vi "Array to Cluster.vi"() -> ()   [LabVIEW 2018]
doc: "Demonstrates the Array to Cluster function."
panel:
  out "Cluster":T1
  in  "Array of Strings":string[](array[string])=["A", "B", "C", "D", "E", "F"]
  # "Overview: Demonstrates the Array to Cluster function.\nInstructions:\n1. Run the VI to convert a portion of the Array of Strings to a Cluster.\n2. Open the block diagram. Right-click on the Array to Cluster function and select Cluster Size from the menu. Change the cluster size to 6.\n3. The VI is now broken because the Cluster indicator does not have six elements.\n4. Delete the Cluster indicator.\n5. On the block diagram, right-click on the output of the Array to Cluster function and select Create > Indicator from the menu. Remove any broken wires.\n6. Run the VI again."
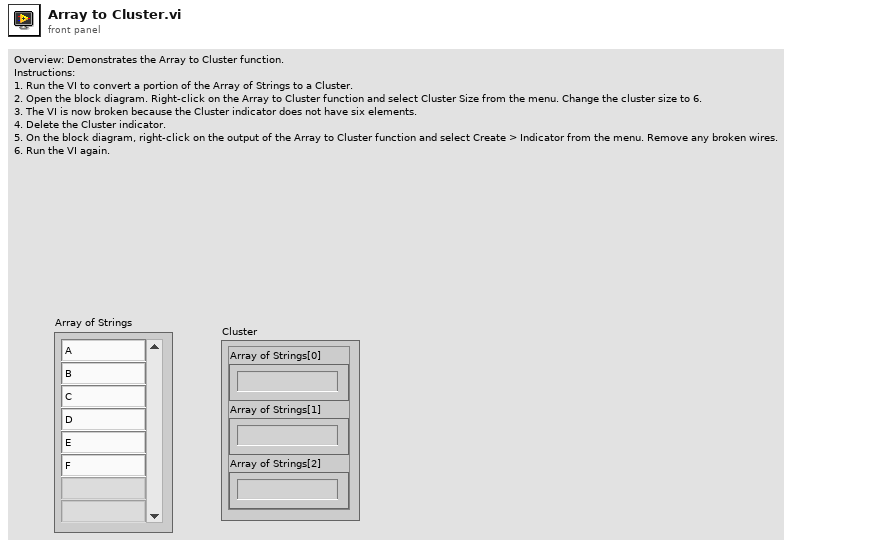
[diagram p1: front panel]
types:
  T1 = cluster{"Array of Strings[0]":string, "Array of Strings[1]":string, "Array of Strings[2]":string}
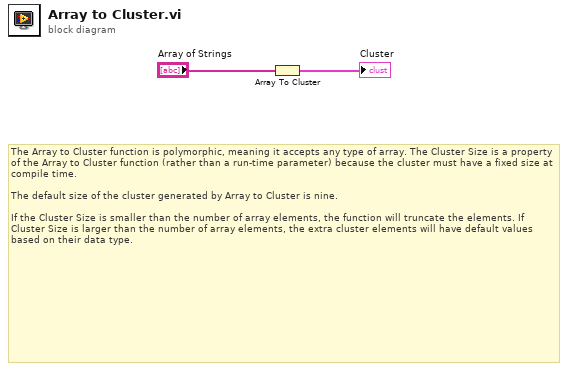
[diagram p0: block diagram]
diagram:
  # "The Array to Cluster function is polymorphic, meaning it accepts any type of array. The Cluster Size is a property of the Array to Cluster function (rather than a run-time parameter) because the cluster must have a fixed size at compile time.\n\nThe default size of the cluster generated by Array to Cluster is nine.\n\nIf the Cluster Size is smaller than the number of array elements, the function will truncate the elements. If Cluster Size is larger than the number of array elements, the extra cluster elements will have default values based on their data type."
  n1 = Array To Cluster(array="Array of Strings") -> (cluster=→"Cluster":T1)
